vi "setUp.vi"(8 "error in (no error)":errorcluster, 11 "reference in":refnum<class "DoNotWaitOnTestComplete.lvclass">) -> (0 "error out":errorcluster, 3 "reference in":refnum<class "DoNotWaitOnTestComplete.lvclass">)   [LabVIEW 2013, in "DoNotWaitOnTestComplete.lvclass"]
uses:
  DoNotWaitOnTestComplete.lvclass
  DoNotWaitOnTestComplete.lvclass/DoNotWaitOnTestComplete.ctl
panel:
  # "Copyright © 2007 James Kring, Inc. All rights reserved.\n\nAuthor: Jim Kring [jim.kring@jameskring.com]\n\nThis library is provided \"AS IS\" ,WITHOUT WARRANTIES OR \nCONDITIONS OF ANY KIND, either express or implied.\n\nJames Kring, Inc. -- http://www.jameskring.com"
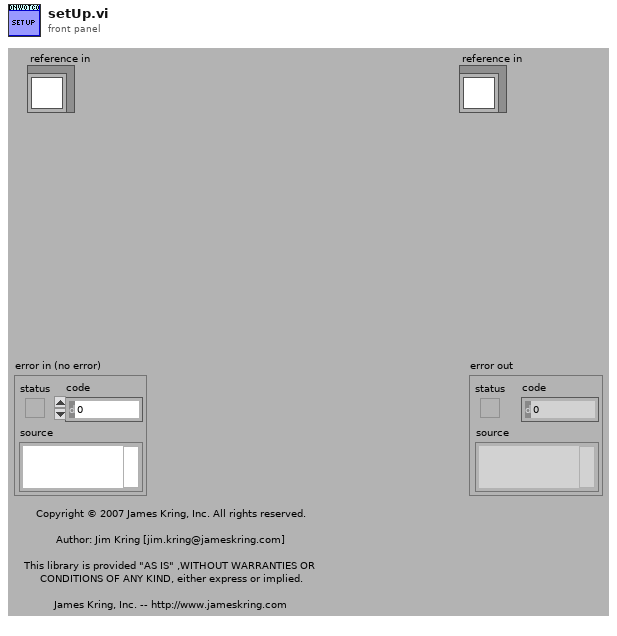
[diagram p1: front panel]
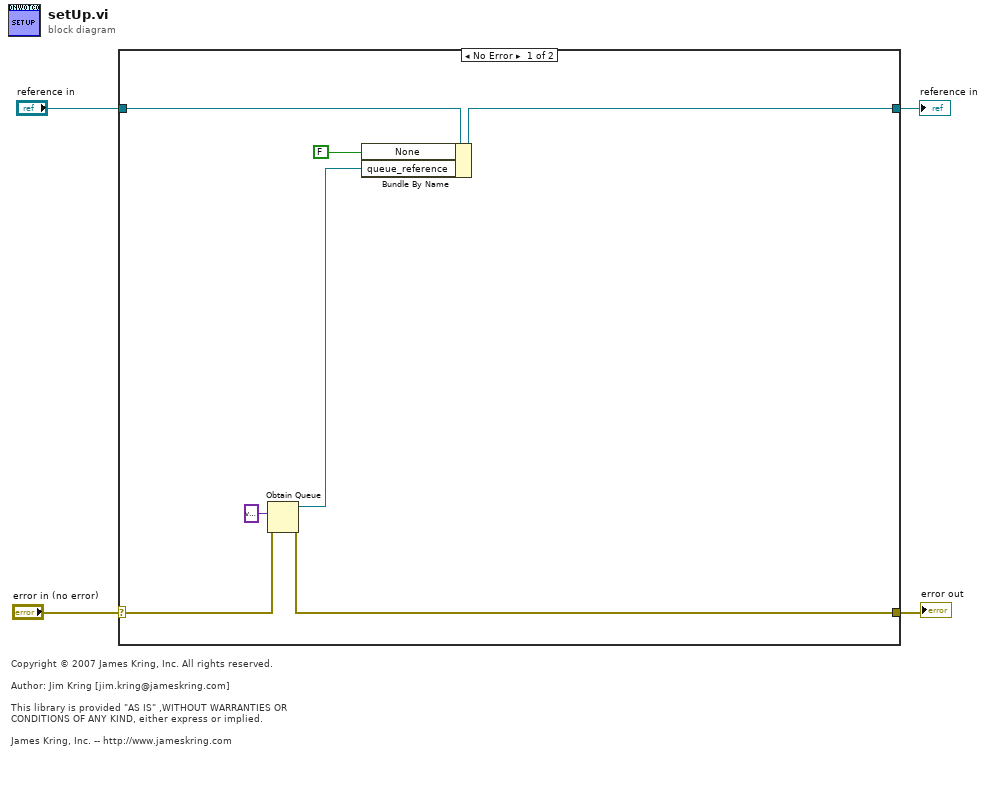
[diagram p0: block diagram]
diagram:
  # "Copyright © 2007 James Kring, Inc. All rights reserved.\n\nAuthor: Jim Kring [jim.kring@jameskring.com]\n\nThis library is provided \"AS IS\" ,WITHOUT WARRANTIES OR \nCONDITIONS OF ANY KIND, either express or implied.\n\nJames Kring, Inc. -- http://www.jameskring.com"
  n1 = case shown="No Error" "error in (no error)" {
    selector: "error in (no error)" -> [w7 w13]
    tunnel: [w6 w13] -> w3
    tunnel: [w5 w12] -> w1
    tunnel: "reference in" -> [w11 w12]
    frame No Error {
      n2 = Obtain Queue(element data type=variant, error in (no error)=w7) -> (queue out=w8:refnum<queue>, error out=w6:errorcluster)  [unwired: 3 in, 1 out]
      n3 = Bundle By Name(cluster=w11, "None"=FALSE, "queue_reference"=w8) -> (w5:refnum<class "DoNotWaitOnTestComplete.lvclass">)
    }
    frame Error {
    }
  }
  "error out" <- w3
  "reference in" <- w1
